vi "Log_PACKET Receive State Machine.vi"(1 "Receive State Machine Local Data":T1 {"Complete Packet"."Packet Data" format="%.0x"}, 11 "Receive State Machine Local Data PREVIOUS":T1 {"Complete Packet"."Packet Data" format="%.0x"}, 12 "error in (no error)":errorcluster, 13 "Command":string) -> (3 "Receive State Machine Local Data dup":T1 {"Complete Packet"."Packet Data" format="%.0x"}, 14 "error out":errorcluster)   [LabVIEW 2014]
uses:
  PacketMode/SRV_PM_Receive State Machine Local Data.ctl
  PacketMode/SRV_PM_Packet.ctl
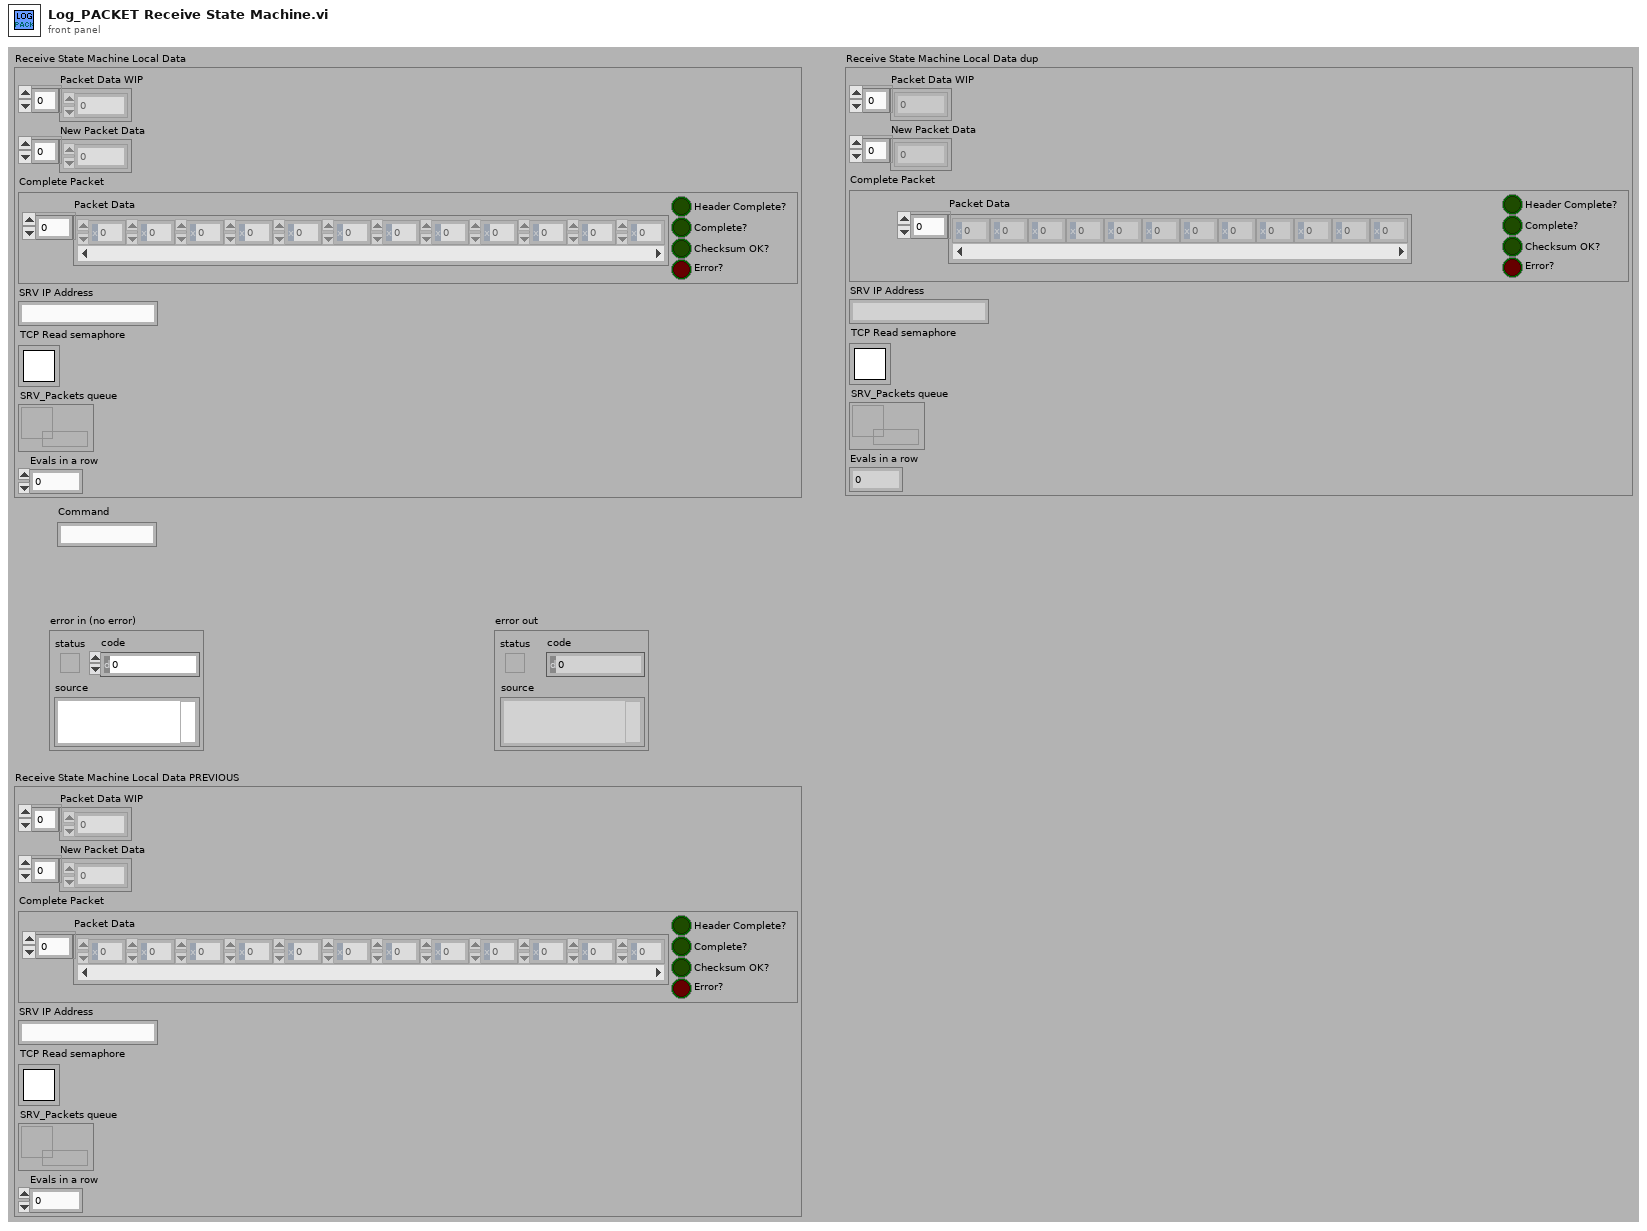
[diagram p1: front panel]
types:
  T1 = typedef "SRV_PM_Receive State Machine Local Data.ctl" = cluster{"Packet Data WIP":u8[], "New Packet Data":u8[], "Complete Packet":T2, "SRV IP Address":string, "TCP Read semaphore":T3, "SRV_Packets queue":refnum<queue>, "Evals in a row":i32}
  T2 = typedef "SRV_PM_Packet.ctl" = cluster{"Packet Data":u8[], "Header Complete?":bool, "Complete?":bool, "Checksum OK?":bool, "Error?":bool}
  T3 = typedef "Semaphore RefNum" = refnum<k1>
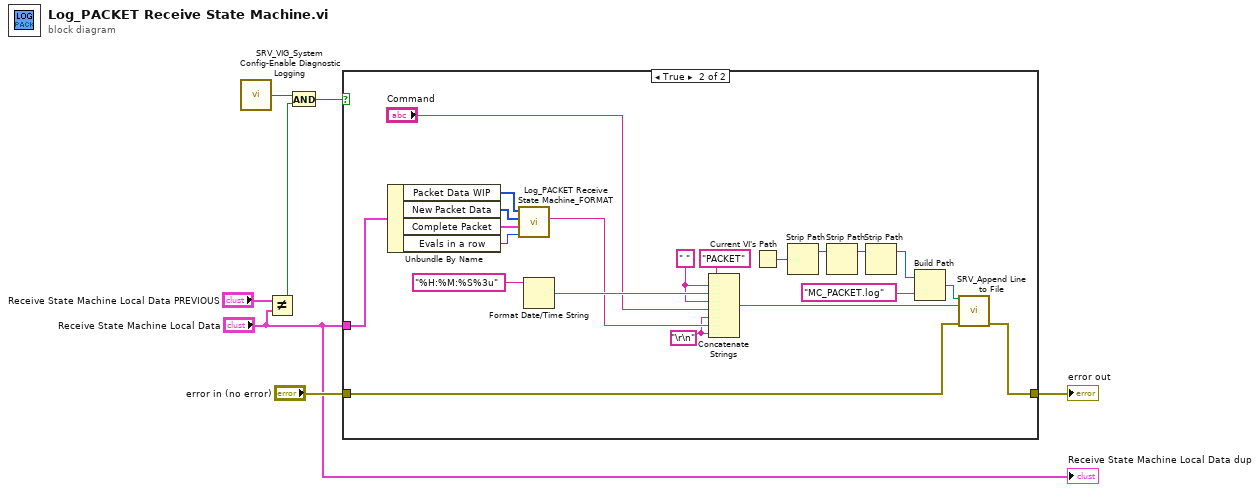
[diagram p0: block diagram]
diagram:
  n1 = call "SRV_VIG_System Config-Enable Diagnostic Logging.vi"() -> ("Enable Diagnostic Log?"=w1:bool)  [unwired: 15 in]
  n2 = Not Equal?(x="Receive State Machine Local Data PREVIOUS", y="Receive State Machine Local Data") -> (x != y?=w2:bool)
  n3 = And(x=w1, y=w2) -> (x .and. y?=w5:bool)
  n4 = case shown="True" w5 {
    tunnel: [w8 w27] -> w7
    tunnel: "error in (no error)" -> [w8 w26]
    tunnel: "Receive State Machine Local Data" -> [_ w16]
    frame False {
    }
    frame True {
      w10 = "\r\n"
      w9 = " " ("string")
      n5 = Unbundle By Name(w16) -> ("Packet Data WIP"=w15:u8[], "New Packet Data"=w14:u8[], "Complete Packet"=w13:T2, "Evals in a row"=w12:i32)
      n6 = call "Log_PACKET Receive State Machine_FORMAT.vi"("Evals in a row"=w12, "Complete Packet"=w13, "New Packet Data"=w14, "Packet Data WIP"=w15) -> ("resulting string"=w11:string)  [unwired: 7 in]
      n7 = Format Date/Time String(time format string (%c)="%H:%M:%S%3u") -> (date/time string=w18:string)  [unwired: 2 in]
      n8 = Concatenate Strings("PACKET" ("string"), w9, w18, w9, "Command", w10, w11, w10) -> (w28:string)
      n9 = Current VI's Path() -> (path=w21:path)
      n10 = Strip Path(path=w21) -> (stripped path=w22:path)  [unwired: 1 out]
      n11 = Strip Path(path=w22) -> (stripped path=w23:path)  [unwired: 1 out]
      n12 = Strip Path(path=w23) -> (stripped path=w20:path)  [unwired: 1 out]
      n13 = Build Path(base path=w20, name or relative path="MC_PACKET.log") -> (appended path=w24:path)
      n14 = call "SRV_Append Line to File.vi"("file path"=w24, "Line to Write"=w28, "error in (no error)"=w26) -> ("error out"=w27:errorcluster)  [unwired: 12 in]
    }
  }
  "error out" <- w7
  "Receive State Machine Local Data dup" <- "Receive State Machine Local Data"
